vi "CAN Get Status.vi"(11 "Channel":u16) -> (3 "function return":u32)   [LabVIEW 2020, in "PCANBasic.lvlib"]
doc: "TPCANStatus __stdcall CAN_GetStatus(\n TPCANHandle Channel);"
uses:
  <userlib>/PCANBasic/PCANBasic.lvlib
  <userlib>/PCANBasic/PCANBasic.dll
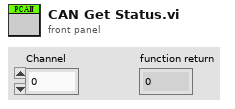
[diagram p1: front panel]
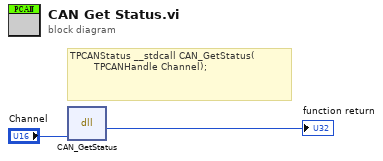
[diagram p0: block diagram]
diagram:
  # "TPCANStatus __stdcall CAN_GetStatus(\n        TPCANHandle Channel);"
  n1 = dll-call lib="D:/Program Files (x86)/National Instruments/LabVIEW 2020/user.lib/PCANBasic/PCANBasic.*" fn="CAN_GetStatus"("Channel"="Channel") -> (→"function return":u32)  [unwired: 4 in, 2 out]
